vi "Close.vi"(8 "error in (no error)":errorcluster, 11 "DMM in":refnum<class "DMM.lvclass">) -> (0 "error out":errorcluster, 2 "Result Text":string="PCI-4070 has been initialized", 3 "DMM out":refnum<class "DMM.lvclass">)   [LabVIEW 2012, in "DMM.lvclass"]
uses:
  DMM.lvclass
  DMM.lvclass/DMM.ctl
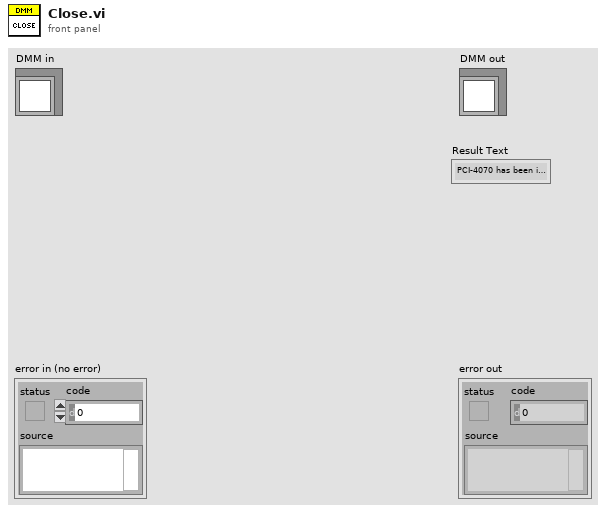
[diagram p1: front panel]
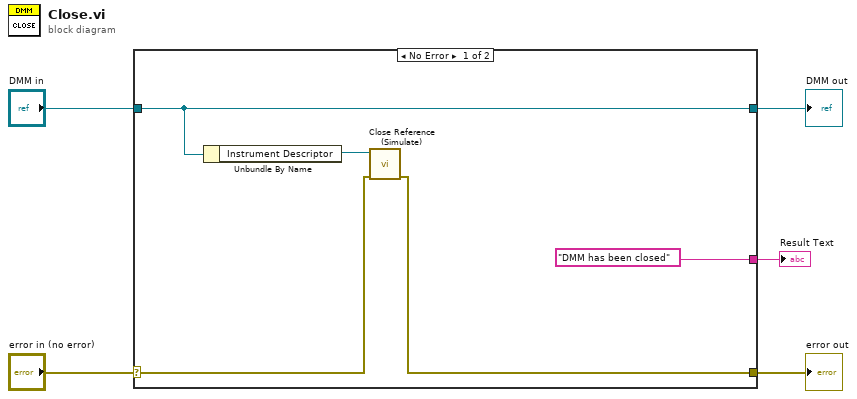
[diagram p0: block diagram]
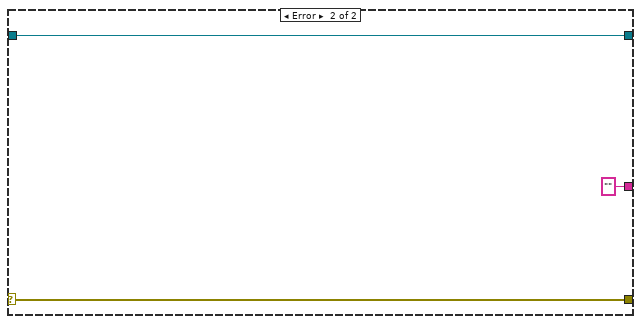
[diagram p2: hidden frame]
diagram:
  n1 = case shown="No Error" "error in (no error)" {
    selector: "error in (no error)" -> [w8 w13]
    tunnel: [w7 w13] -> w4
    tunnel: [w10 w12] -> w2
    tunnel: "DMM in" -> [w10 w12]
    tunnel: ["DMM has been closed" ("Result Text") "" ("Result Text")] -> w1
    frame No Error {
      n2 = Unbundle By Name(w10) -> ("Instrument Descriptor"=w9:refnum<visa-resource-name>)
      n3 = call "Close Reference (Simulate).vi"("error in (no error)"=w8, "Instrument Refnum in"=w9) -> ("error out"=w7:errorcluster)  [unwired: 9 in]
    }
    frame Error {
    }
  }
  "error out" <- w4
  "DMM out" <- w2
  "Result Text" <- w1
